vi "OneShotPulse.vi"(6 "Reset":bool, 11 "Input":bool) -> (2 "Output":bool)   [LabVIEW 2018]
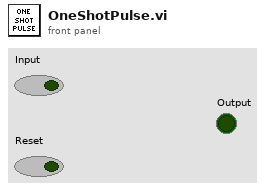
[diagram p1: front panel]
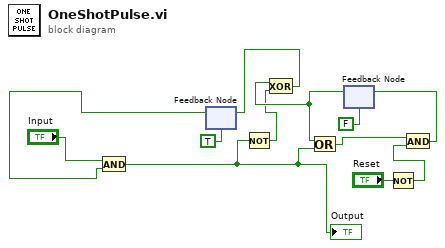
[diagram p0: block diagram]
diagram:
  n1 = feedback #1(TRUE) -> (w10:bool)
  n2 = And(x="Input", y=w10) -> (x .and. y?=w8:bool)
  "Output" <- w8
  n3 = Not(x=w8) -> (.not. x?=w6:bool)
  n4 = feedback #2(FALSE) -> (w7:bool)
  n5 = Exclusive Or(1:w6, 2:w7) -> (0:w5:bool)
  n6 = feedback-in #1(w5) -> ()
  n7 = Or(x=w7, y=w8) -> (x .or. y?=w4:bool)
  n8 = Not(x="Reset") -> (.not. x?=w1:bool)
  n9 = And(x=w4, y=w1) -> (x .and. y?=w3:bool)
  n10 = feedback-in #2(w3) -> ()
